vi "Get Variable Names.vi"(8 "error in (no error)":errorcluster, 11 "Project in":refnum<class "Project.lvclass">) -> (0 "error out":errorcluster, 2 "Variable Names":string[](array[string]), 3 "Project out":refnum<class "Project.lvclass">)   [LabVIEW 2015, in "Project.lvclass"]
uses:
  Project.lvclass
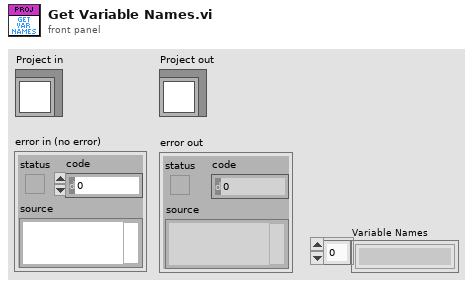
[diagram p1: front panel]
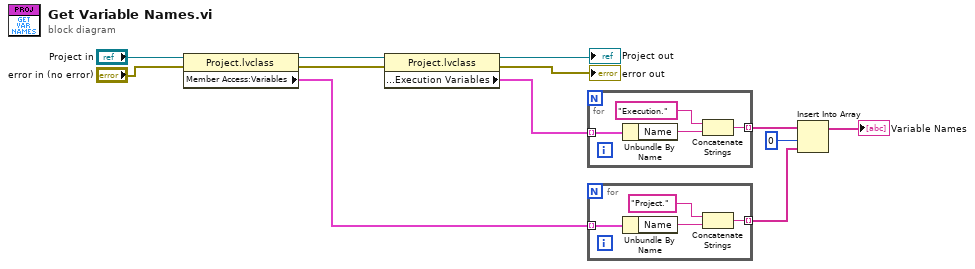
[diagram p0: block diagram]
diagram:
  n1 = property class="Project.lvclass"(reference="Project in", error in="error in (no error)") -> (reference out=w10:refnum<class "Project.lvclass">, error out=w2:errorcluster, "Member Access:Variables"=w11:cluster{"Name":string, "Value":variant}[])
  n2 = property class="Project.lvclass"(reference=w10, error in=w2) -> (reference out=→"Project out":refnum<class "Project.lvclass">, error out=→"error out":errorcluster, "Member Access:Execution Variables"=w9:cluster{"Name":string, "Value":variant}[])
  n3 = for {
    tunnel: w9 -> [w16] mode=indexing
    tunnel: [w13] -> w8 mode=indexing
    n4 = Unbundle By Name(w16) -> ("Name"=w15:string)
    n5 = Concatenate Strings("Execution.", w15) -> (w13:string)
  }
  n6 = for {
    tunnel: w11 -> [w20] mode=indexing
    tunnel: [w17] -> w7 mode=indexing
    n7 = Unbundle By Name(w20) -> ("Name"=w19:string)
    n8 = Concatenate Strings("Project.", w19) -> (w17:string)
  }
  n9 = Insert Into Array(array=w8, index=0, new element=w7) -> (→"Variable Names":string[])
